vi "UHR-Fleezers Control (fpga) - 10.1.vi"() -> ()   [LabVIEW 2009]
doc: "UHR-Fleezers Instrument Control Code (fpga)"
uses:
  <vilib>/Platform/TimedLoop/XDataNode/XDataNode.xnode
  <vilib>/Platform/TimedLoop/XDataNode/loadlvalarms.vi
  <vilib>/Platform/TimedLoop/XDataNode/timing_clust.ctl
  <vilib>/Platform/TimedLoop/XDataNode/nitl_modes.ctl
  <vilib>/Platform/TimedLoop/XDataNode/wakeup.ctl
  <vilib>/eio/EIONode/EIONode.xnode
  <vilib>/rvi/eio/nirviEIOImplementation/nirviEIOImplementation.xnode
  <vilib>/rvi/eio/common/nirviEmuTemplateMethod_noerrors.vi
  <vilib>/rvi/eio/common/nirviEmuClasses.ctl
  <vilib>/eio/EIOMethodNode/EIOMethodNode.xnode
  <vilib>/rvi/eio/nirviEIOMethodImplementation/nirviEIOMethodImplementation.xnode
  <vilib>/rvi/DataTransferAndStorage/Container/XNode/niFpgaContainer.xnode
  <vilib>/rvi/interface/RandomDataEmulation/niFpgaRandomDataHandleErrors.vi
  <vilib>/rvi/interface/RandomDataEmulation/nirviRandomDataFPGAFIFO.vi
  <vilib>/rvi/DataTransferAndStorage/Container/Common/niFpgaContainerMethod.ctl
  <vilib>/rvi/DataTransferAndStorage/Container/Common/niFpgaTransferTypeControl.ctl
  <vilib>/addons/control/pid/fpga.llb/XNode/niFpgaPID.xnode
  <vilib>/Platform/TimedLoop/XDataNode/XDNodeRunTimeDep.lvlib
panel:
  in  "Tab Control":T1(tab)
  in  "AI1 X Scale":u16
  in  "Trap Pos FB Monitor T1 or T2":bool
  in  "Trap Pos FB Negate Action":bool
  in  "Trap Pos. FB SP":fxp<+/-,16,1>
  in  "Trap Pos. FB Reset":bool
  in  "Trap Pos to FIFO":bool
  in  "AI Averages":u16=1 min=1 step=1
  in  "AI1 Sets to FIFO":T2={"Set 1"=TRUE, "Set 2"=TRUE, "Set 3"=FALSE}
  in  "N of AI1 Int Acq Sets":i16=2 min=1 max=3 step=1
  out "Number of AI channels":i16
  out "AI Late Counter":u32
  in  "ai count":u32=400
  out "AI late?":bool
  in  "+ phase":bool
  in  "Phase count adjustment":i16
  out "Relative phase":i16
  in  "DMA buffer timeout":i32
  in  "AI to FIFO":bool
  out "BD1 Frequency Out 1":u64
  out "BD1 Frequency Out 2":u64
  in  "Force feedback":bool
  out "AI1 X Set 1":fxp<+/-,16,1>
  in  "Trap Pos. FB Gains":T3={"proportional gain (Kc)"=0.0, "integral gain (Kc*Ts/Ti)"=10.0, "derivative gain (Kc*Td/Ts)"=0.0} {"proportional gain (Kc)" format="%.11g"; "integral gain (Kc*Ts/Ti)" format="%.11g"; "derivative gain (Kc*Td/Ts)" format="%.11g"}
  in  "Trap Pos. FB Range":T4={"output high"=0.999969482421875, "output low"=-1.0}
  in  "Trap Pos. FB Mult Factor":i64=2
  in  "Trap Pos. FB Offset Factor":i64
  out "AI1 X Set 2":fxp<+/-,16,1>
  out "Trap Pos FB Action":i64
  in  "Tab Control 2":T5(tab)
  in  "Swap F1 and F2":bool
  in  "Freq or Amp switch first":bool=TRUE
  in  "Cont. Scan":bool
  in  "Abort scan":bool
  in  "Cycles per step":u64
  in  "Scan BD":bool
  in  "Number of scans":u16
  in  "Scan steps":u64
  in  "Scan freq.  increment":i64
  out "Scanning":bool
  in  "Start scan":bool
  in  "OSK Bd 1":bool
  in  "Reset Bd 1":bool
  in  "RD":bool
  in  "PMODE":bool
  in  "OSK Bd 2":bool
  in  "Reset Bd 2":bool
  in  "Direct RF Box \nCommunication":bool
  in  "Data BD 2":u8 format="%08b"
  in  "Data BD 1":u8 format="%08b"
  in  "Address":u8 format="%02x"
  in  "Update Data":bool
  in  "FPGA Controls\n RF Box":bool
  in  "Number Interlace Cycles":u8=2 min=1 max=3
  in  "Interlace Off Parameters":u8=1 min=1 max=3
  in  "Interlace ON/OFF":bool
  out "DIO Relative phase":i16
  in  "Phase count adjustment (DIO)":i16
  in  "+ phase (DIO)":bool
  out "DIO Late Counter":u32
  out "DIO Late?":bool
  in  "DIO count 1 (ticks)":u32=400
  in  "DIO count 2 (ticks)":u32=400
  in  "DIO count 3 (ticks)":u32=400
  out "AI2 Y Sum Set 2":i16
  out "AI2 Y Sum Set 1":i16
  in  "FB Gains Set 1":T6={"proportional gain (Kc)"=10, "integral gain (Kc*Ts/Ti)"=5, "derivative gain (Kc*Td/Ts)"=0}
  in  "FB Setpoint Set 1":i16 min=0 step=1
  in  "FB Reset Set 1":bool
  in  "FB On/Off Set 1":bool
  in  "FB Reset Set 2":bool
  in  "FB On/Off Set 2":bool
  in  "FB Setpoint Set 2":i16 min=0 step=1
  in  "FB Gains Set 2":T6={"proportional gain (Kc)"=10, "integral gain (Kc*Ts/Ti)"=5, "derivative gain (Kc*Td/Ts)"=0}
  in  "FB output range 2":cluster{"output high":i16, "output low":i16}={"output high"=3000, "output low"=0}
  in  "FB output range 1":cluster{"output high":i16, "output low":i16}={"output high"=3000, "output low"=0}
  out "Scan I":u64
  in  "Amp switch delay":u16=5
  in  "Freq switch delay":u16
  in  "BD 2 Amplitude 1":u16
  in  "BD 1 Amplitude 1":u16
  in  "BD 2 Frequency 1":u64
  in  "BD 1 Frequency 1":u64
  in  "BD 2 Amplitude 2":u16
  in  "BD 1 Amplitude 2":u16
  in  "BD 2 Frequency 2":u64
  in  "BD 1 Frequency 2":u64
  in  "BD 2 Amplitude 3":u16
  in  "BD 1 Amplitude 3":u16
  in  "BD 2 Frequency 3":u64
  in  "BD 1 Frequency 3":u64
  out "Numeric":i32
  out "AO2 2":i16
  out "AO1 2":i16
  in  "1D or 2D Scan?":bool
  in  "Abort scan (MCL)":bool
  in  "MCL Scan Axis":bool
  in  "Cont. Scan (MCL)":bool
  out "Scan I (MCL)":u64
  in  "Number of scans (MCL)":u16
  out "Scanning MCL":bool
  in  "Scan steps (MCL)":u64
  in  "Cycles per step (MCL)":u64
  in  "Scan freq.  increment (MCL)":i16
  in  "Start scan (MCL)":bool
  in  "AO2":i16
  in  "AO1":i16
  out "MCL Late Counter":u32
  out "MCL Late?":bool
  in  "MCL count":u32=800
  out "MCL Relative Phase":i16
  in  "Phase count adjustment (MCL)":i16
  in  "+ phase (MCL)":bool
  in  "APD2 Trigger on Edge?":bool=TRUE
  in  "APD1 Trigger on Edge?":bool=TRUE
  in  "APD Gate Operating Mode":u8 max=2 step=1
  in  "Invert APD Gate":bool
  in  "APD Gate OFF Count":u32=100
  in  "APD Gate ON Count":u32=300
  out "APD 1 Gate Late Counter":u32
  out "APD 1 Gate Late?":bool
  out "APD 1 Gate Relative Phase":i16
  in  "Phase count adjustment (APD 1 Gate)":i16
  in  "+ phase (APD 1 Gate)":bool
  out "APD 2 Counts 0":u32
  out "APD 2 Counts 1":u32
  out "APD 1 Counts 0":u32
  out "APD 1 Counts 1":u32
  out "APD out state":bool
  in  "APD 2 AO offset":i16
  in  "APD 1 AO offset":i16
  in  "APD 2 AO scale factor":i16=1
  in  "APD 1 AO scale factor":i16=1
  in  "APD to FIFO":bool
  in  "APD Acq Rate Count":u32=20000000
  out "APD Acq Late Counter":u32
  out "APD Acq Late?":bool
  out "APD Acq Relative Phase":i16
  in  "Phase Count Adjustment (APD Acq)":i16
  in  "+ phase (APD Acq)":bool
  in  "Phase count adjustment (APD 2 Gate)":i16
  out "APD 2 Gate Late Counter":u32
  out "APD 2 Gate Late?":bool
  out "APD 2 Gate Relative Phase":i16
  in  "+ phase (APD 2 Gate)":bool
  in  "Green Filter Flipper":bool
  out "Green FB Signals":T7
  in  "Green FB Count":u32=1200
  out "Green Late Counter":u32
  out "Green FB Late?":bool
  out "Green FB Relative Phase":i16
  in  "Phase count adjustment (Green FB)":i16=10
  in  "+ phase (Green FB)":bool
  out "Green FB Sum":i16
  in  "Green int current ON count adj":u32=150
  in  "Current Out":u16=30000
  in  "Green FB On/Off":bool
  in  "Green FB Setpoint":i16=250 min=0 step=1
  in  "Green FB Gains":T6={"proportional gain (Kc)"=10, "integral gain (Kc*Ts/Ti)"=5, "derivative gain (Kc*Td/Ts)"=0}
  in  "Green FB Reset":bool
  in  "Operating Mode 2":u8=2 max=2 step=1
  in  "Invert GI 2":bool
  in  "Green interlace OFF count 2":u32=900
  in  "Green interlace ON count 2":u32=300
  out "GI Late Counter 2":u32
  out "GI Late? 2":bool
  out "GI Relative phase 2":i16
  in  "Phase count adjustment (GI) 2":i16=20
  in  "+ phase (GI) 2":bool
  in  "Green interlace OFF count":u32=100
  out "GI Relative phase":i16
  in  "Phase count adjustment (GI)":i16
  in  "+ phase (GI)":bool
  out "GI Late?":bool
  in  "Green interlace ON count":u32=300
  out "GI Late Counter":u32
  in  "Invert GI":bool
  in  "Operating Mode":u8 max=2 step=1
  in  "Connector0/DIO9":bool
  in  "Connector1/DIO32":bool
  in  "Connector1/DIO33":bool
  in  "Connector1/DIO34":bool
  in  "Chassis2/Mod4/AO1":u16
  in  "Extra DO Counts":u32=40000
  # "Only one of these can be on\nat a time:"
  # "Raster Scan AOD"
  # "1 (X)"
  # "2 (Y)"
  # "IR Intensity Feedback (RF BD 1)"
  # "AO1 (Y)"
  # "2D"
  # "1D"
  # "AO2 (X)"
  # "APD AO for aligning"
  # "Detection Loop"
  # "Green fluorescent laser digital gate interlacing loop"
  # "0 Forced ON\n1 Forced OFF\n2 Interlacing"
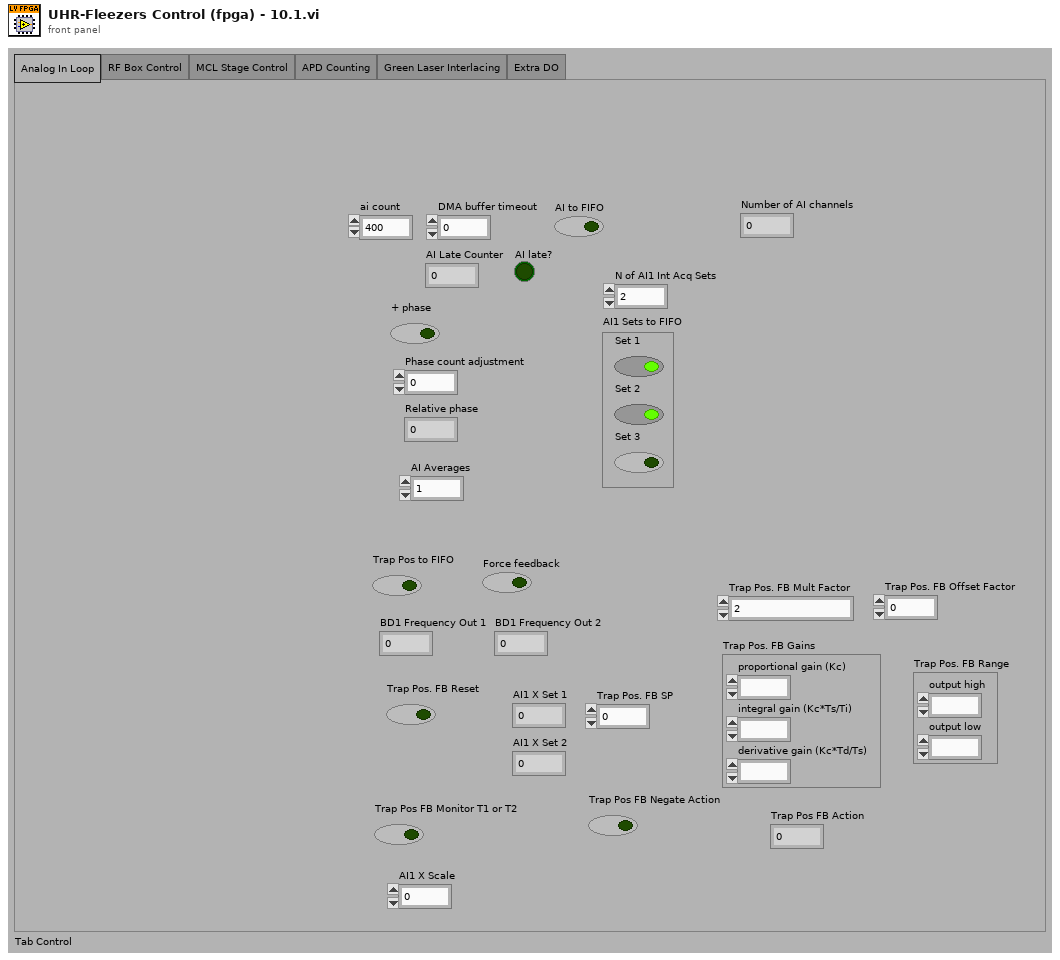
[diagram p1: front panel]
types:
  T1 = enum32{"Analog In Loop", "RF Box Control", "MCL Stage Control", "APD Counting", "Green Laser Interlacing", "Extra DO"}
  T2 = cluster{"Set 1":bool, "Set 2":bool, "Set 3":bool}
  T3 = cluster{"proportional gain (Kc)":fxp<+/-,16,8>, "integral gain (Kc*Ts/Ti)":fxp<+/-,16,8>, "derivative gain (Kc*Td/Ts)":fxp<+/-,16,8>}
  T4 = cluster{"output high":fxp<+/-,16,1>, "output low":fxp<+/-,16,1>}
  T5 = enum32{"Controls", "Interlacing Frequency and Amplitude Values"}
  T6 = cluster{"proportional gain (Kc)":i16, "integral gain (Kc*Ts/Ti)":i16, "derivative gain (Kc*Td/Ts)":i16}
  T7 = cluster{"Green FB Ch 0":i16, "Green FB Ch 1":i16, "Green FB Ch 2":i16}
  T8 = typedef "nirviEmuClasses.ctl" = enum16{"IO Read", "IO Write", "Method", "Property Read", "Property Write"}
  T9 = typedef "XDNodeRunTimeDep.lvlib/timing_clust.ctl" = cluster{"Expected End [f-1]":u64, "Actual End [f-1]":u64, "Finished Late? [f-1]":bool, "Expected End [i-1]":u64, "Actual End [i-1]":u64, "Finished Late? [i-1]":bool, "Expected Start [i]":u64, "Actual Start [i]":u64, "Expected Start [f]":u64, "Actual Start [f]":u64, "Source Name":string, "Structure Name":string, "Period":i64, "Deadline":i64, "Offset":i64, "Start":i64, "Priority":i32, "Timeout":i32, "Mode":T10, "Wakeup Reason":T11, "Error":errorcluster, "Source Type":string, "Secondary Source Type":string, "Global End Time":u64, "Global Start Time":u64, "Frame Duration":u64, "Iteration Duration":u64, "Assigned CPU":i32, "I/O Scan Engine Mode":u32}
  T10 = typedef "XDNodeRunTimeDep.lvlib/nitl_modes.ctl" = enum32{"No Change", "Process missed periods, maintain original phase", "Discard missed periods, maintain original phase", "Process missed periods, ignore original phase", "Discard missed periods, ignore original phase"}
  T11 = typedef "XDNodeRunTimeDep.lvlib/wakeup.ctl" = enum32{"Normal", "Aborted", "Asynchronous wakeup", "Timing source error", "Timed loop error", "Timeout"}
  T12 = typedef "niFpgaContainerMethod.ctl" = enum16{"Write", "Read", "Clear", "Get Number of Elements to Write", "Get Number of Elements to Read", "Enable", "Disable", "Flush and Disable", "Get Stream State"}
  T13 = typedef "niFpgaTransferTypeControl.ctl" = enum16{"Target-Scoped", "Host to Target - DMA", "Target to Host - DMA", "Peer to Peer Reader", "Peer to Peer Writer", "Bidirectional"}
  T14 = cluster{"Chassis2/Mod1/AI0":i16, "Chassis2/Mod1/AI1":i16, "Chassis2/Mod1/AI2":i16}
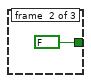
[diagram p2: hidden frame]
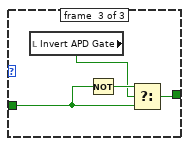
[diagram p3: hidden frame]
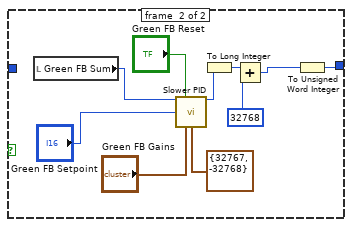
[diagram p4: hidden frame]
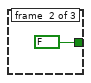
[diagram p5: hidden frame]
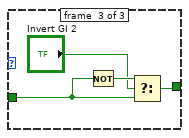
[diagram p6: hidden frame]
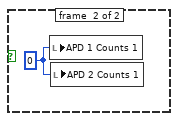
[diagram p7: hidden frame]
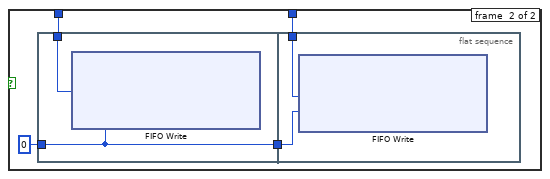
[diagram p8: hidden frame]
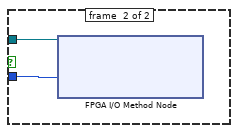
[diagram p9: hidden frame]
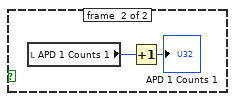
[diagram p10: hidden frame]
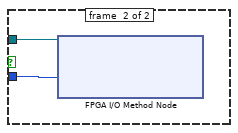
[diagram p11: hidden frame]
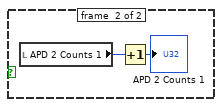
[diagram p12: hidden frame]
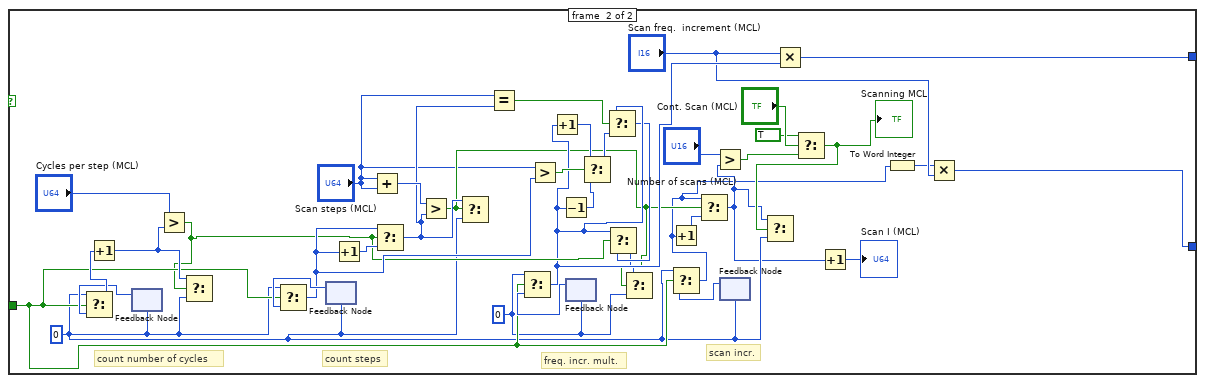
[diagram p13: hidden frame]
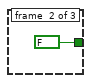
[diagram p14: hidden frame]
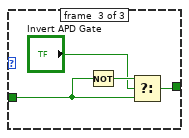
[diagram p15: hidden frame]
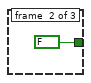
[diagram p16: hidden frame]
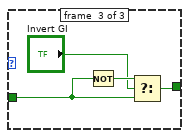
[diagram p17: hidden frame]
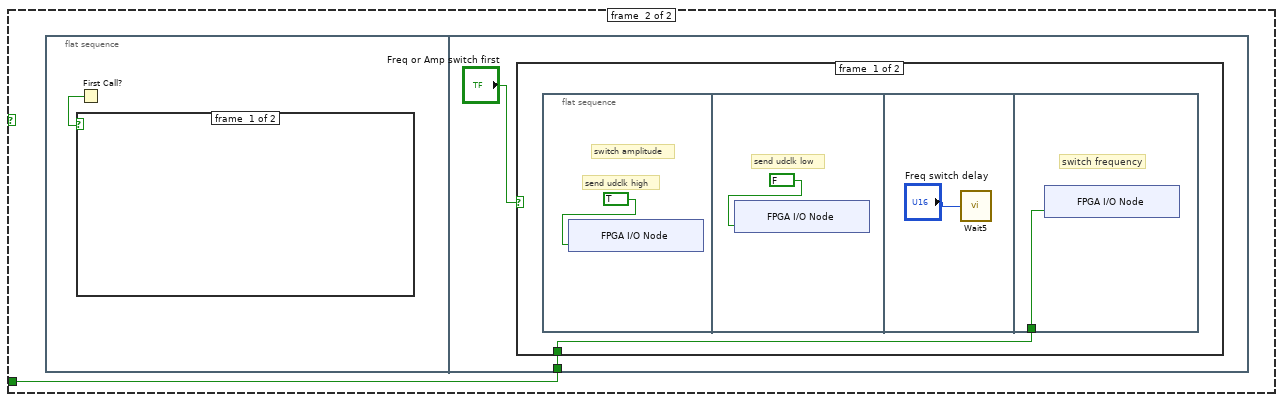
[diagram p18: hidden frame]
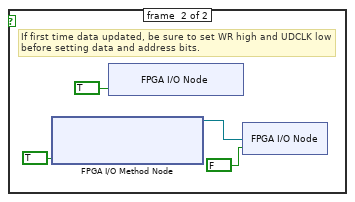
[diagram p19: hidden frame]
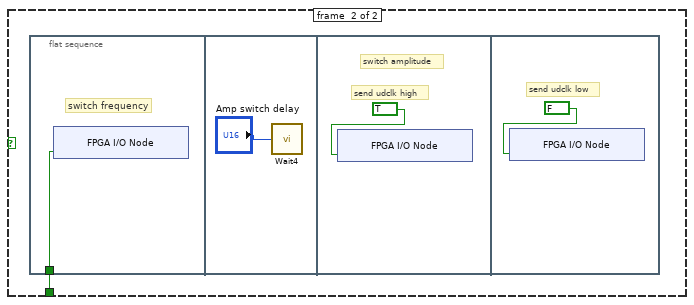
[diagram p20: hidden frame]
diagram:
  w2 = FALSE
  # "timing array current index"
  # "timing array"
  # "timing counter (phase adjusted here)"
  # "late counter"
  n1 = flat-sequence "FPGA initialization to do before running any of the loops" {
    tunnel: [u32 0 ("DIO count 3 (ticks)")] -> w1
    tunnel: [w10] -> _
    frame #0 {
      # "This is a kludge to let host programs know how many channels of data are in the DMA stream.  Set by hand."
      # "Start up expansion chassis early\nto avoid delays later"
      # "This pin controls udclk on the RF boards.\nWhen initially configuring the boards, this pin needs to be\nconfigured as a high impedance input.  Later it will be switched\nto an output."
      # "Initial setting of DIO data and \naddress to low (before reset).  \nThis needs to happen before the other\ncontrol method loops execute."
      n2 = xnode "FPGA I/O Node"("Chassis2/Mod4/AO0"=u16 0) -> ("Chassis2/Mod1/AI0"=w10:i16)  [unwired: 2 in, 2 out]
      n3 = xnode "FPGA I/O Method Node"("Enable"=FALSE) -> ()  [unwired: 1 in, 1 out]
      n4 = xnode "FPGA I/O Node"("Connector1/DIO0"=FALSE, "Connector1/DIO1"=FALSE, "Connector1/DIO2"=FALSE, "Connector1/DIO3"=FALSE, "Connector1/DIO4"=FALSE, "Connector1/DIO5"=FALSE, "Connector1/DIO6"=FALSE, "Connector1/DIO7"=FALSE, "Connector1/DIO8"=FALSE, "Connector1/DIO9"=FALSE, "Connector1/DIO10"=FALSE, "Connector1/DIO11"=FALSE, "Connector1/DIO12"=FALSE, "Connector1/DIO13"=FALSE, "Connector1/DIO15"=FALSE, "Connector1/DIO20"=FALSE, "Connector1/DIO21"=FALSE, "Connector1/DIO22"=FALSE, "Connector1/DIO23"=FALSE, "Connector1/DIO24"=FALSE, "Connector1/DIO25"=FALSE, "Connector1/DIO26"=FALSE, "Connector1/DIO27"=FALSE, "Connector1/DIO14"=FALSE) -> ()  [unwired: 24 in, 24 out]
      "Number of AI channels" <- i16 12 ("Number of AI channels")
    }
  }
  n5 = local read "AO1"() -> (w6:i16)
  n6 = local read "AO2"() -> (w5:i16)
  n7 = node-c288() -> (w4:T9)  [unwired: 1 in]
  n8 = while "APD 1 Counter" {
    tunnel: w1 -> [_]
    stop <- FALSE stop-if-true
    n9 = flat-sequence {
      frame #0 {
        n10 = case shown="False" "APD1 Trigger on Edge?" {
          tunnel: refnum<k21> "Connector0/DIO0" ("APD 1 DO") -> [w398 w423]
          tunnel: -1 ("Timeout") -> [w397 w422]
          frame #0 {
            n11 = xnode "FPGA I/O Method Node"("FPGA I/O In"=w398, "Timeout"=w397) -> ()  [unwired: 2 out]
          }
          frame #1 {
            n12 = xnode "FPGA I/O Method Node"("FPGA I/O In"=w423, "Timeout"=w422) -> ()  [unwired: 2 out]
          }
        }
      }
      frame #1 {
        n13 = local read "APD out state"() -> (w447:bool)
        n14 = case shown="False" w447 {
          frame #0 {
            n15 = local read "APD 1 Counts 0"() -> (w449:u32)
            n16 = Increment(x=w449) -> (x+1=→"APD 1 Counts 0":u32)
          }
          frame #1 {
            n17 = local read "APD 1 Counts 1"() -> (w451:u32)
            n18 = Increment(x=w451) -> (x+1=→"APD 1 Counts 1":u32)
          }
        }
      }
    }
  }
  n19 = while "APD 2 Counter" {
    tunnel: w1 -> [_]
    stop <- FALSE stop-if-true
    n20 = flat-sequence {
      frame #0 {
        n21 = case shown="False" "APD2 Trigger on Edge?" {
          tunnel: refnum<k21> "Connector0/DIO1" ("APD 2 DO") -> [w457 w482]
          tunnel: -1 ("Timeout") -> [w456 w481]
          frame #0 {
            n22 = xnode "FPGA I/O Method Node"("FPGA I/O In"=w457, "Timeout"=w456) -> ()  [unwired: 2 out]
          }
          frame #1 {
            n23 = xnode "FPGA I/O Method Node"("FPGA I/O In"=w482, "Timeout"=w481) -> ()  [unwired: 2 out]
          }
        }
      }
      frame #1 {
        n24 = local read "APD out state"() -> (w506:bool)
        n25 = case shown="False" w506 {
          frame #0 {
            n26 = local read "APD 2 Counts 0"() -> (w508:u32)
            n27 = Increment(x=w508) -> (x+1=→"APD 2 Counts 0":u32)
          }
          frame #1 {
            n28 = local read "APD 2 Counts 1"() -> (w510:u32)
            n29 = Increment(x=w510) -> (x+1=→"APD 2 Counts 1":u32)
          }
        }
      }
    }
  }
  n30 = while "APD 2 Gating" {
    shift-right: [w514] -> _
    shift-left: w1 -> [w519]
    shift-right: [w513] -> _
    shift-left: w2 -> [w511]
    stop <- FALSE stop-if-true
    n31 = flat-sequence {
      tunnel: w519 -> [w522]
      tunnel: [w523] -> w517
      tunnel: [w522] -> w515
      tunnel: [w521] -> w512
      tunnel: w511 -> [w521]
      tunnel: [w526] -> w518
      tunnel: w517 -> [w526]
      tunnel: [w525] -> w516
      tunnel: w515 -> [w525]
      tunnel: w512 -> [w524]
      tunnel: [w580] -> w514
      tunnel: w518 -> [w598]
      tunnel: w516 -> [w596]
      tunnel: [w585] -> w513
      frame #0 {
        n32 = call "Loop Timer8"("Count(Ticks)"=w522) -> ("Tick Count(Ticks)"=w523:u32)
      }
      frame #1 {
        # "(need 4 channels/APD)"
        n33 = xnode "FPGA I/O Node"("Connector0/DIO8"=w524, "Connector0/DIO9"=w524, "Connector0/DIO10"=w524, "Connector0/DIO11"=w524) -> ()  [unwired: 4 in, 4 out]
      }
      frame #2 {
        n34 = local read "APD Gate ON Count"() -> (w573:u32)
        n35 = local read "APD Gate OFF Count"() -> (w572:u32)
        n36 = feedback #1(TRUE) -> (w587:bool)
        n37 = feedback #2(w598) -> (w574:u32)
        n38 = Not(x=w587) -> (.not. x?=w584:bool)
        n39 = Subtract(x=w598, y=w574) -> (x-y=w597:u32)
        n40 = Select(t=w573, s=w584, f=w572) -> (s? t:f=w589:u32)
        n41 = Subtract(x=w597, y=w596) -> (x-y=w590:u32)
        n42 = Subtract(x=w589, y=w590) -> (x-y=w579:u32)
        n43 = Greater?(x=w590, y=u32 0) -> (0:w592:bool)
        "APD 2 Gate Late?" <- w592
        n44 = Boolean To (0,1)(Boolean="+ phase (APD 2 Gate)") -> (0, 1=w577:i16)
        n45 = Multiply(x=w577, y="Phase count adjustment (APD 2 Gate)") -> (x*y=w575:i16)
        n46 = feedback #3(u32 0) -> (w594:u32)
        n47 = Increment(x=w594) -> (x+1=w593:u32)
        n48 = Select(t=w593, s=w592, f=w594) -> (s? t:f=w591:u32)
        "APD 2 Gate Late Counter" <- w591
        n49 = Add(x=w579, y=w575) -> (x+y=w580:u32)
        n50 = feedback #4(i16 0) -> (w582:i16)
        n51 = Subtract(x=w582, y=w575) -> (x-y=w581:i16)
        "APD 2 Gate Relative Phase" <- w581
        n52 = local read "APD Gate Operating Mode"() -> (w571:u8)
        n53 = case shown="2" w571 {
          tunnel: [TRUE FALSE w604] -> w585
          tunnel: w587 -> [_ _ w602]
          frame #0 {
          }
          frame #1 {
          }
          frame #2 {
            n54 = local read "Invert APD Gate"() -> (w601:bool)
            n55 = Not(x=w602) -> (.not. x?=w603:bool)
            n56 = Select(t=w603, s=w601, f=w602) -> (s? t:f=w604:bool)
          }
        }
      }
    }
  }
  n57 = while "DAQ AI set 1" {
    shift-right: [w605] -> _
    shift-left: w1 -> [w610]
    stop <- FALSE stop-if-true
    n58 = flat-sequence {
      tunnel: w610 -> [w620]
      tunnel: [w621] -> w608
      tunnel: [w620] -> w607
      tunnel: [w631] -> w618
      tunnel: [w630] -> w617
      tunnel: [w629] -> w616
      tunnel: [w628] -> w615
      tunnel: [w627] -> w614
      tunnel: [w626] -> w613
      tunnel: [w625] -> w612
      tunnel: [w624] -> w611
      tunnel: [w623] -> w609
      tunnel: w608 -> [w623]
      tunnel: w607 -> [w622]
      tunnel: [w622] -> w606
      tunnel: [w817] -> w605
      tunnel: w618 -> [w852]
      tunnel: w617 -> [w808]
      tunnel: w616 -> [w809]
      tunnel: w615 -> [w851]
      tunnel: w614 -> [w840]
      tunnel: w613 -> [w839]
      tunnel: w612 -> [w838]
      tunnel: w611 -> [w837]
      tunnel: w609 -> [w834]
      tunnel: w606 -> [w831]
      frame #0 {
        n59 = call "Loop Timer3"("Count(Ticks)"=w620) -> ("Tick Count(Ticks)"=w621:u32)
      }
      frame #1 {
        n60 = xnode "FPGA I/O Node"("Connector1/DIO31"=TRUE ("Connector1/DIO33")) -> ("Connector0/AI0"=w631:i16, "Connector0/AI1"=w630:i16, "Connector0/AI2"=w629:i16, "Connector0/AI3"=w628:i16, "Connector0/AI4"=w627:i16, "Connector0/AI5"=w626:i16, "Connector0/AI6"=w625:i16, "Connector0/AI7"=w624:i16)  [unwired: 9 in, 9 out]
      }
      frame #2 {
        w812 = FALSE ("AI to FIFO")
        # "Adjust phase after data acquired if button pressed"
        n61 = feedback #5(i16 1) -> (w844:i16)
        n62 = Increment(x=w844) -> (x+1=w850:i16)
        n63 = Scale By Power Of 2(n="AI1 X Scale", x=w808) -> (x*2^n=w806:i16)
        n64 = Greater?(x=w850, y="N of AI1 Int Acq Sets") -> (0:w847:bool)
        n65 = Divide(x=w806, y=w809) -> (x/y=w805:fxp<+/-,16,1>)
        n66 = Select(t=i16 1, s=w847, f=w850) -> (s? t:f=w849:i16)
        n67 = feedback #6(w812) -> (w810:bool)
        n68 = feedback #7(w812) -> (w836:bool)
        n69 = case shown="1, Default" w844 {
          tunnel: w809 -> [w855 w890 _]
          tunnel: "AI1 Sets to FIFO" -> [w861 w896 w927]
          tunnel: [w859 w894 w926] -> w841
          tunnel: ["AI to FIFO" w893 w925] -> w835
          tunnel: w836 -> [_ w893 w925]
          tunnel: "DMA buffer timeout" -> [w860 w895 _]
          tunnel: ["Trap Pos to FIFO" w891 w924] -> w811
          tunnel: w810 -> [_ w891 w924]
          tunnel: w805 -> [w854 w889 _]
          frame #0 {
            n70 = Unbundle By Name(w861) -> ("Set 1"=w859:bool)
            n71 = Compound Arithmetic op=AND("Trap Pos to FIFO", w859, "AI to FIFO") -> (w857:bool)
            n72 = case shown="True" w857 {
              tunnel: w860 -> [_ w863]
              frame #0 {
              }
              frame #1 {
                n73 = local read "BD1 Frequency Out 1"() -> (w862:u64)
                n74 = xnode ("FIFO Method Node")("Element"=w862, "Timeout"=w863) -> ()  [unwired: 1 in, 2 out]
              }
            }
            "AI2 Y Sum Set 1" <- w855
            "AI1 X Set 1" <- w854
          }
          frame #1 {
            n75 = Unbundle By Name(w896) -> ("Set 2"=w894:bool)
            n76 = Compound Arithmetic op=AND(w891, w894, w893) -> (w892:bool)
            n77 = case shown="True" w892 {
              tunnel: w895 -> [_ w898]
              frame #0 {
              }
              frame #1 {
                n78 = local read "BD1 Frequency Out 2"() -> (w897:u64)
                n79 = xnode ("FIFO Method Node")("Element"=w897, "Timeout"=w898) -> ()  [unwired: 1 in, 2 out]
              }
            }
            "AI2 Y Sum Set 2" <- w890
            "AI1 X Set 2" <- w889
          }
          frame #2 {
            n80 = Unbundle By Name(w927) -> ("Set 3"=w926:bool)
          }
        }
        n81 = And(x=w841, y=w835) -> (x .and. y?=w843:bool)
        n82 = case shown="True" w843 {
          tunnel: w852 -> [_ w932]
          tunnel: w808 -> [_ w933]
          tunnel: w809 -> [_ w934]
          tunnel: w851 -> [_ w935]
          tunnel: w840 -> [_ w939]
          tunnel: w839 -> [_ w938]
          tunnel: w838 -> [_ w937]
          tunnel: w837 -> [_ w936]
          tunnel: "DMA buffer timeout" -> [_ w928]
          frame #0 {
          }
          frame #1 {
            n83 = Greater?(x="AI Averages", y=u16 1) -> (0:w930:bool)
            n84 = case shown="False" w930 {
              tunnel: w939 -> [w950 w1007]
              tunnel: w938 -> [w949 w1006]
              tunnel: w937 -> [w948 w1005]
              tunnel: w936 -> [w947 w1004]
              tunnel: w935 -> [w946 w1003]
              tunnel: w934 -> [w951 w1002]
              tunnel: w933 -> [w952 w1001]
              tunnel: w932 -> [w953 w1000]
              tunnel: "AI Averages" -> [_ w987]
              tunnel: w928 -> [w941 w984]
              frame #0 {
                n85 = Join Numbers(hi=w953, lo=w952) -> ((hi.lo)=w945:u32)
                n86 = Join Numbers(hi=w951, lo=w946) -> ((hi.lo)=w944:u32)
                n87 = Join Numbers(hi=w950, lo=w949) -> ((hi.lo)=w943:u32)
                n88 = Join Numbers(hi=w948, lo=w947) -> ((hi.lo)=w942:u32)
                n89 = Build Array(w945, w944, w943, w942) -> (w940:u32[])
                n90 = for {
                  tunnel: w940 -> [w955] mode=indexing
                  tunnel: w941 -> [w956]
                  n91 = To Unsigned Long Integer(number=w955) -> (unsigned 32bit integer=w954:u32)
                  n92 = xnode ("FIFO Write")("Element"=w954, "Timeout"=w956) -> ()  [unwired: 1 in, 2 out]
                }
              }
              frame #1 {
                w991 = u16 0
                n93 = To Long Integer(number=w1000) -> (32bit integer=w993:i32)
                n94 = To Long Integer(number=w1001) -> (32bit integer=w1010:i32)
                n95 = To Long Integer(number=w1002) -> (32bit integer=w1009:i32)
                n96 = To Long Integer(number=w1003) -> (32bit integer=w1008:i32)
                n97 = To Long Integer(number=w1007) -> (32bit integer=w999:i32)
                n98 = To Long Integer(number=w1006) -> (32bit integer=w998:i32)
                n99 = To Long Integer(number=w1005) -> (32bit integer=w997:i32)
                n100 = To Long Integer(number=w1004) -> (32bit integer=w996:i32)
                n101 = Build Array(w993, w1010, w1009, w1008, w999, w998, w997, w996) -> (w982:i32[])
                n102 = feedback #8(w982) -> (w995:i32[])
                n103 = Add(x=w982, y=w995) -> (x+y=w994:i32[])
                n104 = feedback #9(w991) -> (w989:u16)
                n105 = Increment(x=w989) -> (x+1=w986:u16)
                n106 = Equal?(x=w986, y=u16 1) -> (x = y?=w985:bool)
                n107 = Select(t=w982, s=w985, f=w994) -> (s? t:f=w983:i32[])
                n108 = Greater Or Equal?(x=w986, y=w987) -> (x >= y?=w988:bool)
                n109 = Select(t=w991, s=w988, f=w986) -> (s? t:f=w990:u16)
                n110 = case shown="True" w988 {
                  tunnel: w983 -> [_ w1012]
                  tunnel: w984 -> [_ w1011]
                  frame #0 {
                  }
                  frame #1 {
                    n111 = for {
                      tunnel: w1012 -> [w1014] mode=indexing
                      tunnel: w1011 -> [w1015]
                      n112 = To Unsigned Long Integer(number=w1014) -> (unsigned 32bit integer=w1013:u32)
                      n113 = xnode ("FIFO Write")("Element"=w1013, "Timeout"=w1015) -> ()  [unwired: 1 in, 2 out]
                    }
                  }
                }
              }
            }
          }
        }
        n114 = feedback #10(w834) -> (w833:u32)
        n115 = Subtract(x=w834, y=w833) -> (x-y=w832:u32)
        n116 = Subtract(x=w832, y=w831) -> (x-y=w828:u32)
        n117 = Subtract(x="ai count", y=w828) -> (x-y=w818:u32)
        n118 = Greater?(x=w828, y=u32 0) -> (0:w826:bool)
        "AI late?" <- w826
        n119 = xnode "I/O Node"("Connector1/DIO31"=FALSE ("Connector1/DIO34")) -> ()  [unwired: 1 in, 1 out]
        n120 = Boolean To (0,1)(Boolean="+ phase") -> (0, 1=w820:i16)
        n121 = feedback #11(u32 0) -> (w824:u32)
        n122 = Increment(x=w824) -> (x+1=w823:u32)
        n123 = Select(t=w823, s=w826, f=w824) -> (s? t:f=w825:u32)
        "AI Late Counter" <- w825
        n124 = Multiply(x=w820, y="Phase count adjustment") -> (x*y=w814:i16)
        n125 = feedback #12(i16 0) -> (w816:i16)
        n126 = Add(x=w818, y=w814) -> (x+y=w817:u32)
        n127 = Subtract(x=w816, y=w814) -> (x-y=w815:i16)
        "Relative phase" <- w815
      }
    }
  }
  n128 = while "RF box board DIO control: parallel communication" {
    shift-right: [w1060] -> _
    shift-left: w1 -> [w1059]
    shift-right: [w1058] -> _
    shift-left: FALSE ("Swap F1 and F2") -> [w1057]
    stop <- FALSE stop-if-true
    n129 = flat-sequence {
      tunnel: w1057 -> [w1064]
      tunnel: w1059 -> [w1062]
      tunnel: [w1064] -> w1056
      tunnel: [w1063] -> w1055
      tunnel: [w1062] -> w1054
      tunnel: [w1070] -> w1060
      tunnel: [w1069] -> w1058
      tunnel: w1056 -> [w1068]
      tunnel: w1055 -> [w1066]
      tunnel: w1054 -> [w1065]
      frame #0 {
        n130 = call "Loop Timer"("Count(Ticks)"=w1062) -> ("Tick Count(Ticks)"=w1063:u32)
      }
      frame #1 {
        n131 = flat-sequence {
          tunnel: ["FPGA Controls\n RF Box"] -> w1067
          tunnel: w1068 -> [w1071]
          tunnel: [w1220] -> w1070
          tunnel: [w1240] -> w1069
          tunnel: w1067 -> [w1239]
          tunnel: w1066 -> [w1233]
          tunnel: w1065 -> [w1230]
          frame #0 {
            n132 = case shown="True" "FPGA Controls\n RF Box" {
              tunnel: w1071 -> [_ w1073]
              frame #0 {
              }
              frame #1 {
                n133 = flat-sequence {
                  tunnel: w1073 -> [w1118]
                  frame #0 {
                    n134 = First Call?() -> (First Call?: T/F=w1074:bool)
                    n135 = case shown="True" w1074 {
                      frame #0 {
                      }
                      frame #1 {
                        # "If first time data updated, be sure to set WR high and UDCLK low\nbefore setting data and address bits."
                        n136 = xnode "FPGA I/O Method Node"("Enable"=TRUE) -> ("FPGA I/O Out"=w1076:refnum<k21>)  [unwired: 1 in]
                        n137 = xnode "FPGA I/O Node"("Connector1/DIO15"=TRUE) -> ()  [unwired: 1 in, 1 out]
                        n138 = xnode "FPGA I/O Node"("I/O Item"=FALSE ("Connector1/DIO30"), "FPGA I/O In"=w1076) -> ()  [unwired: 1 out]
                      }
                    }
                  }
                  frame #1 {
                    n139 = case shown="True" "Freq or Amp switch first" {
                      tunnel: w1118 -> [w1120 w1164]
                      frame #0 {
                        n140 = flat-sequence {
                          tunnel: w1120 -> [w1150]
                          frame #0 {
                            # "switch amplitude"
                            # "send udclk high"
                            n141 = xnode "FPGA I/O Node"("Connector1/DIO30"=TRUE ("Connector1/DIO15")) -> ()  [unwired: 1 in, 1 out]
                          }
                          frame #1 {
                            # "send udclk low"
                            n142 = xnode "FPGA I/O Node"("Connector1/DIO30"=FALSE ("Connector1/DIO15")) -> ()  [unwired: 1 in, 1 out]
                          }
                          frame #2 {
                            n143 = call "Wait5"("Count(Ticks)"="Freq switch delay") -> ()  [unwired: 1 out]
                          }
                          frame #3 {
                            # "switch frequency"
                            n144 = xnode "FPGA I/O Node"("Connector1/DIO36"=w1150) -> ()  [unwired: 1 in, 1 out]
                          }
                        }
                      }
                      frame #1 {
                        n145 = flat-sequence {
                          tunnel: w1164 -> [w1165]
                          frame #0 {
                            # "switch frequency"
                            n146 = xnode "FPGA I/O Node"("Connector1/DIO36"=w1165) -> ()  [unwired: 1 in, 1 out]
                          }
                          frame #1 {
                            n147 = call "Wait4"("Count(Ticks)"="Amp switch delay") -> ()  [unwired: 1 out]
                          }
                          frame #2 {
                            # "switch amplitude"
                            # "send udclk high"
                            n148 = xnode "FPGA I/O Node"("Connector1/DIO30"=TRUE ("Connector1/DIO15")) -> ()  [unwired: 1 in, 1 out]
                          }
                          frame #3 {
                            # "send udclk low"
                            n149 = xnode "FPGA I/O Node"("Connector1/DIO30"=FALSE ("Connector1/DIO15")) -> ()  [unwired: 1 in, 1 out]
                          }
                        }
                      }
                    }
                  }
                }
              }
            }
          }
          frame #1 {
            # "This is the prior cycle's on time"
            # "increment timing\nindex, reset to 0 if \nend of matrix"
            # "Reset to begginning (1) when number of cycles reached."
            # "timing index"
            # "build byte stacks for writing data\n(must correspond to addresses array constant)"
            # "Timing housekeeping"
            # "Adjust phase if late\n(maintains constant phase relationship between cycles)"
            n150 = feedback #13(u8 0 ("t")) -> (w1236:u8)
            n151 = Increment(x=w1236) -> (x+1=w1280:u8)
            n152 = Increment(x="Number Interlace Cycles") -> (x+1=w1275:u8)
            n153 = Equal?(x=w1280, y=w1275) -> (x = y?=w1282:bool)
            n154 = Select(t=u8 1, s=w1282, f=w1280) -> (s? t:f=w1235:u8)
            n155 = Increment(x=w1235) -> (x+1=w1277:u8)
            n156 = Equal?(x=w1277, y=w1275) -> (x = y?=w1278:bool)
            n157 = Select(t=u8 1, s=w1278, f=w1277) -> (s? t:f=w1274:u8)
            n158 = Select(t=w1274, s="Interlace ON/OFF", f="Interlace Off Parameters") -> (s? t:f=w1258:u8)
            n159 = case shown="1, Default" w1258 {
              tunnel: [w1357 "BD 1 Frequency 2" "BD 1 Frequency 3"] -> w1270
              tunnel: [w1356 "BD 2 Frequency 2" "BD 2 Frequency 3"] -> w1259
              tunnel: ["BD 2 Amplitude 1" "BD 2 Amplitude 2" "BD 2 Amplitude 3"] -> w1208
              tunnel: [w1345 w1473 "BD 1 Amplitude 3"] -> w1211
              frame #0 {
                w1352 = u64 0 ("f")
                # "Trap 1"
                n160 = local read "Scanning"() -> (w1358:bool)
                n161 = Or(x=w1358, y="Start scan") -> (x .or. y?=w1350:bool)
                n162 = Not(x="Abort scan") -> (.not. x?=w1348:bool)
                n163 = And(x=w1348, y=w1350) -> (x .and. y?=w1347:bool)
                n164 = case "For raster scanning" shown="False" w1347 {
                  tunnel: [u64 0 w1461] -> w1353
                  tunnel: "Start scan" -> [_ w1446]
                  frame #0 {
                    n165 = local write "Scanning"(FALSE ("scanning")) -> ()
                  }
                  frame #1 {
                    w1430 = i64 0
                    w1429 = u64 0
                    # "scan incr."
                    # "freq. incr. mult."
                    # "count steps"
                    # "count number of cycles"
                    n166 = feedback #14(w1429) -> (w1458:u64)
                    n167 = Select(t=w1429, s=w1446, f=w1458) -> (s? t:f=w1460:u64)
                    n168 = Increment(x=w1460) -> (x+1=w1457:u64)
                    n169 = Greater?(x="Cycles per step", y=w1457) -> (0:w1439:bool)
                    n170 = Select(t=w1457, s=w1439, f=w1429) -> (s? t:f=w1456:u64)
                    n171 = feedback #15(w1429) -> (w1455:u64)
                    n172 = Select(t=w1429, s=w1446, f=w1455) -> (s? t:f=w1450:u64)
                    n173 = Increment(x=w1450) -> (x+1=w1454:u64)
                    n174 = Add(x="Scan steps", y="Scan steps") -> (x+y=w1453:u64)
                    n175 = Select(t=w1450, s=w1439, f=w1454) -> (s? t:f=w1434:u64)
                    n176 = Greater?(x=w1453, y=w1434) -> (0:w1433:bool)
                    n177 = Select(t=w1434, s=w1433, f=w1429) -> (s? t:f=w1451:u64)
                    n178 = Equal?(x="Scan steps", y=w1434) -> (x = y?=w1438:bool)
                    n179 = Greater?(x="Scan steps", y=w1450) -> (0:w1449:bool)
                    n180 = feedback #16(w1430) -> (w1452:i64)
                    n181 = Select(t=w1430, s=w1446, f=w1452) -> (s? t:f=w1436:i64)
                    n182 = Increment(x=w1436) -> (x+1=w1448:i64)
                    n183 = Decrement(x=w1436) -> (x-1=w1447:i64)
                    n184 = Select(t=w1448, s=w1449, f=w1447) -> (s? t:f=w1437:i64)
                    n185 = Select(t=w1436, s=w1438, f=w1437) -> (s? t:f=w1435:i64)
                    n186 = Select(t=w1436, s=w1439, f=w1435) -> (s? t:f=w1431:i64)
                    n187 = Select(t=w1431, s=w1433, f=w1430) -> (s? t:f=w1432:i64)
                    n188 = feedback #17(w1429) -> (w1445:u64)
                    n189 = Select(t=w1429, s=w1446, f=w1445) -> (s? t:f=w1441:u64)
                    n190 = Increment(x=w1441) -> (x+1=w1442:u64)
                    n191 = Select(t=w1441, s=w1433, f=w1442) -> (s? t:f=w1440:u64)
                    n192 = Greater?(x="Number of scans", y=w1440) -> (0:w1426:bool)
                    n193 = Multiply(x="Scan freq.  increment", y=w1436) -> (x*y=w1461:i64)
                    n194 = Select(t=TRUE, s="Cont. Scan", f=w1426) -> (s? t:f=w1425:bool)
                    "Scanning" <- w1425
                    n195 = Select(t=w1440, s=w1425, f=w1429) -> (s? t:f=w1443:u64)
                    n196 = Increment(x=w1440) -> (x+1=→"Scan I":u64)
                  }
                }
                n197 = case "For position feedback" shown="True" "Force feedback" {
                  tunnel: [i64 0 w1376] -> w1342
                  frame #0 {
                  }
                  frame #1 {
                    n198 = case shown="False" "Trap Pos FB Monitor T1 or T2" {
                      tunnel: [w1383 w1384] -> w1370
                      frame #0 {
                        n199 = local read "AI1 X Set 2"() -> (w1383:fxp<+/-,16,1>)
                      }
                      frame #1 {
                        n200 = local read "AI1 X Set 1"() -> (w1384:fxp<+/-,16,1>)
                      }
                    }
                    n201 = xnode ("PID")("process variable"=w1370, "reset?"="Trap Pos. FB Reset", "setpoint"="Trap Pos. FB SP", "PID gains"="Trap Pos. FB Gains", "output range"="Trap Pos. FB Range") -> ("output"=w1374:fxp<+/-,16,1>)
                    n202 = Negate(x=w1374) -> (-x=w1373:fxp<+/-,17,2>)
                    n203 = Select(t=w1373, s="Trap Pos FB Negate Action", f=w1374) -> (s? t:f=w1368:fxp<+/-,17,2>)
                    n204 = Scale By Power Of 2(n=u32 15, x=u32 1) -> (x*2^n=w1365:u32)
                    n205 = Multiply(x=w1368, y=w1365) -> (x*y=w1364:fxp<+/-,17,17>)
                    n206 = To Quad Integer(1:w1364) -> (0:w1379:i64)
                    "Trap Pos FB Action" <- w1379
                    n207 = Multiply(x=w1379, y="Trap Pos. FB Mult Factor") -> (x*y=w1377:i64)
                    n208 = Add(x=w1377, y="Trap Pos. FB Offset Factor") -> (x+y=w1376:i64)
                  }
                }
                n209 = case "For intensity feedback" shown="True" "FB On/Off Set 1" {
                  tunnel: "BD 1 Amplitude 1" -> [w1463 _]
                  tunnel: [w1463 w1464] -> w1345
                  frame #0 {
                  }
                  frame #1 {
                    n210 = local read "AI2 Y Sum Set 1"() -> (w1466:i16)
                    n211 = call "Slower PID.vi"("process variable"=w1466, "reset?"="FB Reset Set 1", "setpoint"="FB Setpoint Set 1", "PID gains (x 2^8)"="FB Gains Set 1", "output range"="FB output range 1") -> ("output"=w1469:i16)  [unwired: 10 out]
                    n212 = To Unsigned Word Integer(number=w1469) -> (unsigned 16bit integer=w1464:u16)
                  }
                }
                n213 = Select(t=w1352, s="Scan BD", f=w1353) -> (s? t:f=w1351:u64)
                n214 = Select(t=w1353, s="Scan BD", f=w1352) -> (s? t:f=w1354:u64)
                n215 = Add(x=w1351, y="BD 2 Frequency 1") -> (x+y=w1356:u64)
                n216 = Compound Arithmetic op=ADD("BD 1 Frequency 1", w1342, w1354) -> (w1357:u64)
                "BD1 Frequency Out 1" <- w1357
              }
              frame #1 {
                # "Trap 2"
                n217 = case shown="True" "FB On/Off Set 2" {
                  tunnel: [w1477 w1478] -> w1473
                  tunnel: "BD 1 Amplitude 2" -> [w1477 _]
                  frame #0 {
                  }
                  frame #1 {
                    n218 = local read "AI2 Y Sum Set 2"() -> (w1483:i16)
                    n219 = call "Slower PID.vi"("process variable"=w1483, "reset?"="FB Reset Set 2", "setpoint"="FB Setpoint Set 2", "PID gains (x 2^8)"="FB Gains Set 2", "output range"="FB output range 2") -> ("output"=w1480:i16)  [unwired: 10 out]
                    n220 = To Unsigned Word Integer(number=w1480) -> (unsigned 16bit integer=w1478:u16)
                  }
                }
                "BD1 Frequency Out 2" <- "BD 1 Frequency 2"
              }
              frame #2 {
                # "Fluorescence period"
              }
            }
            n221 = feedback #18(w1233) -> (w1232:u32)
            n222 = Subtract(x=w1233, y=w1232) -> (x-y=w1231:u32)
            n223 = Select(t=w1235, s="Interlace ON/OFF", f="Interlace Off Parameters") -> (s? t:f=w1273:u8)
            n224 = Subtract "The error"(x=w1231, y=w1230) -> (x-y=w1228:u32)
            n225 = case shown="3" w1273 {
              tunnel: ["DIO count 1 (ticks)" "DIO count 2 (ticks)" "DIO count 3 (ticks)"] -> w1229
              frame #0 {
              }
              frame #1 {
              }
              frame #2 {
              }
            }
            n226 = Greater?(x=w1228, y=u32 0) -> (0:w1223:bool)
            "DIO Late?" <- w1223
            n227 = feedback #19(u32 0) -> (w1225:u32)
            n228 = Increment(x=w1225) -> (x+1=w1224:u32)
            n229 = Select(t=w1224, s=w1223, f=w1225) -> (s? t:f=w1226:u32)
            "DIO Late Counter" <- w1226
            n230 = Subtract(x=w1229, y=w1228) -> (x-y=w1221:u32)
            n231 = Boolean To (0,1)(Boolean="+ phase (DIO)") -> (0, 1=w1218:i16)
            n232 = Multiply(x=w1218, y="Phase count adjustment (DIO)") -> (x*y=w1214:i16)
            n233 = feedback #20(i16 0) -> (w1216:i16)
            n234 = Subtract(x=w1216, y=w1214) -> (x-y=w1215:i16)
            "DIO Relative phase" <- w1215
            n235 = Split Number(x=w1270) -> (hi(x)=w1269:u32, lo(x)=w1268:u32)
            n236 = Split Number(x=w1259) -> (hi(x)=w1264:u32, lo(x)=w1263:u32)
            n237 = Split Number(x=w1269) -> (lo(x)=w1267:u16)  [unwired: 1 out]
            n238 = Split Number(x=w1268) -> (hi(x)=w1266:u16, lo(x)=w1265:u16)
            n239 = Split Number(x=w1264) -> (lo(x)=w1262:u16)  [unwired: 1 out]
            n240 = Split Number(x=w1263) -> (hi(x)=w1261:u16, lo(x)=w1260:u16)
            n241 = Split Number(x=w1211) -> (hi(x)=w1213:u8, lo(x)=w1212:u8)
            n242 = Split Number(x=w1208) -> (hi(x)=w1210:u8, lo(x)=w1209:u8)
            n243 = Add(x=w1221, y=w1214) -> (x+y=w1220:u32)
            n244 = Split Number(x=w1267) -> (hi(x)=w1257:u8, lo(x)=w1256:u8)
            n245 = Split Number(x=w1266) -> (hi(x)=w1255:u8, lo(x)=w1254:u8)
            n246 = Split Number(x=w1262) -> (hi(x)=w1250:u8, lo(x)=w1249:u8)
            n247 = Split Number(x=w1265) -> (hi(x)=w1253:u8, lo(x)=w1252:u8)
            n248 = Split Number(x=w1261) -> (hi(x)=w1248:u8, lo(x)=w1247:u8)
            n249 = Split Number(x=w1260) -> (hi(x)=w1246:u8, lo(x)=w1245:u8)
            n250 = Build Array "BD 1 A Stack"(w1213, w1212) -> (w1242:u8[])
            n251 = Build Array "BD 2 A Stack"(w1210, w1209) -> (w1241:u8[])
            n252 = Build Array "BD 1 nu Stack"(w1257, w1256, w1255, w1254, w1253, w1252) -> (w1251:u8[])
            n253 = Build Array "BD 2 nu Stack"(w1250, w1249, w1248, w1247, w1246, w1245) -> (w1244:u8[])
            n254 = case shown="2" w1258 {
              tunnel: [w1334 w1337] -> w1240
              tunnel: [u8 10 u8 4] -> w1243
              tunnel: "Swap F1 and F2" -> [w1335 w1337]
              frame #0 {
                # "F2"
                n255 = Not(x=w1335) -> (.not. x?=w1334:bool)
              }
              frame #1 {
                # "low chooses F1"
                # "F1"
              }
            }
            n256 = case "If FPGA is controlling (toggling) RF synth" shown="True" w1239 {
              tunnel: w1251 -> [_ w1287]
              tunnel: w1244 -> [_ w1286]
              tunnel: w1243 -> [_ w1285]
              tunnel: w1242 -> [_ w1284]
              tunnel: w1241 -> [_ w1283]
              frame #0 {
              }
              frame #1 {
                # "Write next amp.\n(wait until beginning of next loop iteration to update)"
                n257 = flat-sequence "Update the next F1 and F2 frequency value (the actual frequency won't change until FSK is switched).\nThen load the next amplitude value into buffer, but don't update it until the next cycle." {
                  tunnel: w1287 -> [w1290]
                  tunnel: w1286 -> [w1289]
                  tunnel: w1285 -> [w1288]
                  tunnel: w1284 -> [w1327]
                  tunnel: w1283 -> [w1326]
                  frame #0 {
                    n258 = for {
                      tunnel: w1290 -> [w1296] mode=indexing
                      tunnel: w1289 -> [w1295] mode=indexing
                      tunnel: w1288 -> [w1293]
                      i -> [w1294]
                      # "Write next freq."
                      n259 = To Unsigned Byte Integer(number=w1294) -> (unsigned 8bit integer=w1291:u8)
                      n260 = Add(x=w1293, y=w1291) -> (x+y=w1292:u8)
                      n261 = call "write to RF synth bd.vi"("Address Byte"=w1292, "BD 2 Byte"=w1295, "BD 1 Byte"=w1296) -> ()
                    }
                  }
                  frame #1 {
                    # "send udclk high"
                    n262 = xnode "FPGA I/O Node"("Connector1/DIO30"=TRUE ("Connector1/DIO15")) -> ()  [unwired: 1 in, 1 out]
                  }
                  frame #2 {
                    n263 = xnode "FPGA I/O Node"("Connector1/DIO30"=FALSE ("Connector1/DIO15")) -> ()  [unwired: 1 in, 1 out]
                  }
                  frame #3 {
                    n264 = for {
                      tunnel: w1327 -> [w1333] mode=indexing
                      tunnel: w1326 -> [w1332] mode=indexing
                      tunnel: u8 33 -> [w1330]
                      i -> [w1331]
                      n265 = To Unsigned Byte Integer(number=w1331) -> (unsigned 8bit integer=w1328:u8)
                      n266 = Add(x=w1330, y=w1328) -> (x+y=w1329:u8)
                      n267 = call "write to RF synth bd.vi"("Address Byte"=w1329, "BD 2 Byte"=w1332, "BD 1 Byte"=w1333) -> ()
                    }
                  }
                }
              }
            }
          }
        }
      }
    }
  }
  n268 = while "MCL stage control" {
    shift-right: [w1504] -> _
    shift-left: w1 -> [w1507]
    shift-right: [w1497] -> _
    shift-left: w6 -> [w1494]
    shift-right: [w1496] -> _
    shift-left: w5 -> [w1492]
    i -> [w1491]
    stop <- FALSE stop-if-true
    n269 = flat-sequence {
      tunnel: w1507 -> [w1511]
      tunnel: [w1512] -> w1503
      tunnel: [w1511] -> w1501
      tunnel: [w1510] -> w1495
      tunnel: w1494 -> [w1510]
      tunnel: [w1509] -> w1493
      tunnel: w1492 -> [w1509]
      tunnel: w1503 -> [w1516]
      tunnel: [w1516] -> w1502
      tunnel: w1501 -> [w1515]
      tunnel: [w1515] -> w1500
      tunnel: w1495 -> [w1514]
      tunnel: w1493 -> [w1513]
      tunnel: [w1514] -> w1490
      tunnel: [w1513] -> w1489
      tunnel: w1502 -> [w1550]
      tunnel: w1500 -> [w1549]
      tunnel: [w1550] -> w1506
      tunnel: [w1549] -> w1505
      tunnel: [w1548] -> w1499
      tunnel: [w1547] -> w1498
      tunnel: w1490 -> [w1542]
      tunnel: w1489 -> [w1541]
      tunnel: [w1614] -> w1504
      tunnel: w1506 -> [w1628]
      tunnel: w1505 -> [w1625]
      tunnel: w1499 -> [w1617]
      tunnel: w1498 -> [w1616]
      tunnel: [w1617] -> w1497
      tunnel: [w1616] -> w1496
      frame #0 {
        n270 = call "Loop Timer5"("Count(Ticks)"=w1511) -> ("Tick Count(Ticks)"=w1512:u32)
      }
      frame #1 {
        n271 = xnode "FPGA I/O Node"("Connector0/AO1"=w1514, "Connector0/AO2"=w1513) -> ()  [unwired: 2 in, 2 out]
      }
      frame #2 {
        n272 = local read "Scanning MCL"() -> (w1562:bool)
        n273 = Or(x=w1562, y="Start scan (MCL)") -> (x .or. y?=w1557:bool)
        n274 = Not(x="Abort scan (MCL)") -> (.not. x?=w1555:bool)
        n275 = And(x=w1555, y=w1557) -> (x .and. y?=w1554:bool)
        n276 = case "Raster scan" shown="True" w1554 {
          tunnel: [w1563 w1606] -> w1559
          tunnel: "Start scan (MCL)" -> [_ w1591]
          tunnel: [w1563 w1567] -> w1543
          frame #0 {
            w1563 = i16 0
            n277 = local write "Scanning MCL"(FALSE ("scanning")) -> ()
          }
          frame #1 {
            w1577 = i16 0
            w1576 = u64 0
            # "scan incr."
            # "freq. incr. mult."
            # "count steps"
            # "count number of cycles"
            n278 = feedback #21(w1576) -> (w1603:u64)
            n279 = Select(t=w1576, s=w1591, f=w1603) -> (s? t:f=w1605:u64)
            n280 = Increment(x=w1605) -> (x+1=w1602:u64)
            n281 = Greater?(x="Cycles per step (MCL)", y=w1602) -> (0:w1586:bool)
            n282 = Select(t=w1602, s=w1586, f=w1576) -> (s? t:f=w1601:u64)
            n283 = feedback #22(w1576) -> (w1600:u64)
            n284 = Select(t=w1576, s=w1591, f=w1600) -> (s? t:f=w1595:u64)
            n285 = Increment(x=w1595) -> (x+1=w1599:u64)
            n286 = Add(x="Scan steps (MCL)", y="Scan steps (MCL)") -> (x+y=w1598:u64)
            n287 = Select(t=w1595, s=w1586, f=w1599) -> (s? t:f=w1581:u64)
            n288 = Greater?(x=w1598, y=w1581) -> (0:w1580:bool)
            n289 = Select(t=w1581, s=w1580, f=w1576) -> (s? t:f=w1596:u64)
            n290 = Equal?(x="Scan steps (MCL)", y=w1581) -> (x = y?=w1585:bool)
            n291 = Greater?(x="Scan steps (MCL)", y=w1595) -> (0:w1594:bool)
            n292 = feedback #23(w1577) -> (w1597:i16)
            n293 = Select(t=w1577, s=w1591, f=w1597) -> (s? t:f=w1583:i16)
            n294 = Increment(x=w1583) -> (x+1=w1593:i16)
            n295 = Decrement(x=w1583) -> (x-1=w1592:i16)
            n296 = Select(t=w1593, s=w1594, f=w1592) -> (s? t:f=w1584:i16)
            n297 = Select(t=w1583, s=w1585, f=w1584) -> (s? t:f=w1582:i16)
            n298 = Select(t=w1583, s=w1586, f=w1582) -> (s? t:f=w1578:i16)
            n299 = Select(t=w1578, s=w1580, f=w1577) -> (s? t:f=w1579:i16)
            n300 = feedback #24(w1576) -> (w1590:u64)
            n301 = Select(t=w1576, s=w1591, f=w1590) -> (s? t:f=w1565:u64)
            n302 = Increment(x=w1565) -> (x+1=w1587:u64)
            n303 = Select(t=w1565, s=w1580, f=w1587) -> (s? t:f=w1566:u64)
            n304 = Greater?(x="Number of scans (MCL)", y=w1566) -> (0:w1573:bool)
            n305 = Multiply(x="Scan freq.  increment (MCL)", y=w1583) -> (x*y=w1606:i16)
            n306 = Select(t=TRUE, s="Cont. Scan (MCL)", f=w1573) -> (s? t:f=w1572:bool)
            "Scanning MCL" <- w1572
            n307 = Select(t=w1566, s=w1572, f=w1576) -> (s? t:f=w1588:u64)
            n308 = Increment(x=w1566) -> (x+1=→"Scan I (MCL)":u64)
            n309 = To Word Integer(number=w1565) -> (16bit integer=w1568:i16)
            n310 = Multiply(x=w1568, y="Scan freq.  increment (MCL)") -> (x*y=w1567:i16)
          }
        }
        n311 = Select(t=w1543, s="1D or 2D Scan?", f=i16 0) -> (s? t:f=w1544:i16)
        n312 = Select(t=w1544, s="MCL Scan Axis", f=w1559) -> (s? t:f=w1558:i16)
        n313 = Select(t=w1559, s="MCL Scan Axis", f=w1544) -> (s? t:f=w1560:i16)
        n314 = Add(x=w1558, y="AO2") -> (x+y=w1547:i16)
        n315 = Add(x="AO1", y=w1560) -> (x+y=w1548:i16)
        "AO1 2" <- w1542
        "AO2 2" <- w1541
      }
      frame #3 {
        n316 = feedback #25(w1628) -> (w1627:u32)
        n317 = Boolean To (0,1)(Boolean="+ phase (MCL)") -> (0, 1=w1612:i16)
        n318 = Subtract(x=w1628, y=w1627) -> (x-y=w1626:u32)
        n319 = Multiply(x=w1612, y="Phase count adjustment (MCL)") -> (x*y=w1608:i16)
        n320 = Subtract(x=w1626, y=w1625) -> (x-y=w1623:u32)
        n321 = Subtract(x="MCL count", y=w1623) -> (x-y=w1610:u32)
        n322 = feedback #26(i16 0) -> (w1609:i16)
        n323 = Subtract(x=w1609, y=w1608) -> (x-y=w1607:i16)
        "MCL Relative Phase" <- w1607
        n324 = Greater?(x=w1623, y=u32 0) -> (0:w1622:bool)
        "MCL Late?" <- w1622
        n325 = Add(x=w1610, y=w1608) -> (x+y=w1614:u32)
        n326 = feedback #27(u32 0) -> (w1620:u32)
        n327 = Increment(x=w1620) -> (x+1=w1619:u32)
        n328 = Select(t=w1619, s=w1622, f=w1620) -> (s? t:f=w1621:u32)
        "MCL Late Counter" <- w1621
      }
    }
    "Numeric" <- w1491
  }
  n329 = while "APD 1 Gating" {
    shift-right: [w1633] -> _
    shift-left: w1 -> [w1638]
    shift-right: [w1632] -> _
    shift-left: w2 -> [w1630]
    stop <- FALSE stop-if-true
    n330 = flat-sequence {
      tunnel: w1638 -> [w1641]
      tunnel: [w1642] -> w1636
      tunnel: [w1641] -> w1634
      tunnel: [w1640] -> w1631
      tunnel: w1630 -> [w1640]
      tunnel: [w1645] -> w1637
      tunnel: w1636 -> [w1645]
      tunnel: [w1644] -> w1635
      tunnel: w1634 -> [w1644]
      tunnel: w1631 -> [w1643]
      tunnel: [w1695] -> w1633
      tunnel: w1637 -> [w1717]
      tunnel: w1635 -> [w1714]
      tunnel: [w1700] -> w1632
      frame #0 {
        n331 = call "Loop Timer7"("Count(Ticks)"=w1641) -> ("Tick Count(Ticks)"=w1642:u32)
      }
      frame #1 {
        # "(need 4 channels/APD)"
        n332 = xnode "FPGA I/O Node"("Connector0/DIO4"=w1643, "Connector0/DIO5"=w1643, "Connector0/DIO6"=w1643, "Connector0/DIO7"=w1643) -> ()  [unwired: 4 in, 4 out]
      }
      frame #2 {
        n333 = feedback #28(TRUE) -> (w1703:bool)
        n334 = feedback #29(w1717) -> (w1716:u32)
        n335 = Not(x=w1703) -> (.not. x?=w1699:bool)
        n336 = Subtract(x=w1717, y=w1716) -> (x-y=w1715:u32)
        n337 = Select(t="APD Gate ON Count", s=w1699, f="APD Gate OFF Count") -> (s? t:f=w1705:u32)
        n338 = Subtract(x=w1715, y=w1714) -> (x-y=w1706:u32)
        n339 = Subtract(x=w1705, y=w1706) -> (x-y=w1694:u32)
        n340 = Greater?(x=w1706, y=u32 0) -> (0:w1710:bool)
        "APD 1 Gate Late?" <- w1710
        n341 = Boolean To (0,1)(Boolean="+ phase (APD 1 Gate)") -> (0, 1=w1692:i16)
        n342 = Multiply(x=w1692, y="Phase count adjustment (APD 1 Gate)") -> (x*y=w1690:i16)
        n343 = feedback #30(u32 0) -> (w1712:u32)
        n344 = Increment(x=w1712) -> (x+1=w1711:u32)
        n345 = Select(t=w1711, s=w1710, f=w1712) -> (s? t:f=w1709:u32)
        "APD 1 Gate Late Counter" <- w1709
        n346 = Add(x=w1694, y=w1690) -> (x+y=w1695:u32)
        n347 = feedback #31(i16 0) -> (w1697:i16)
        n348 = Subtract(x=w1697, y=w1690) -> (x-y=w1696:i16)
        "APD 1 Gate Relative Phase" <- w1696
        n349 = case shown="2" "APD Gate Operating Mode" {
          tunnel: [TRUE FALSE w1723] -> w1700
          tunnel: w1703 -> [_ _ w1720]
          frame #0 {
          }
          frame #1 {
          }
          frame #2 {
            n350 = Not(x=w1720) -> (.not. x?=w1722:bool)
            n351 = Select(t=w1722, s="Invert APD Gate", f=w1720) -> (s? t:f=w1723:bool)
          }
        }
      }
    }
  }
  n352 = while "RF box board direct communication loop" {
    tunnel: w1 -> [_]
    stop <- FALSE stop-if-true
    n353 = case "Whether to use direct communication method (only use one method at a time)" shown="True" "Direct RF Box \nCommunication" {
      frame #0 {
      }
      frame #1 {
        n354 = case shown="True" "Update Data" {
          frame #0 {
          }
          frame #1 {
            n355 = flat-sequence {
              frame #0 {
                n356 = First Call?() -> (First Call?: T/F=w1727:bool)
                n357 = case shown="True" w1727 {
                  frame #0 {
                  }
                  frame #1 {
                    # "If first time data updated, be sure to set WR high\nbefore setting data and address bits."
                    n358 = flat-sequence {
                      frame #0 {
                        n359 = xnode "FPGA I/O Node"("Connector1/DIO15"=TRUE) -> ()  [unwired: 1 in, 1 out]
                      }
                      frame #1 {
                        n360 = call "Wait"("Count(Ticks)"=u8 40 ("DO Delay 3 (Ticks)")) -> ()  [unwired: 1 out]
                      }
                    }
                  }
                }
              }
              frame #1 {
                n361 = Number To Boolean Array(number="Address") -> (Boolean array=w1789:bool[])
                n362 = Number To Boolean Array(number="Data BD 1") -> (Boolean array=w1790:bool[])
                n363 = Number To Boolean Array(number="Data BD 2") -> (Boolean array=w1759:bool[])
                n364 = Index Array(array=w1790, index=7) -> (element=w1774:bool)
                n365 = Index Array(array=w1790, index=6) -> (element=w1773:bool)
                n366 = Index Array(array=w1790, index=5) -> (element=w1772:bool)
                n367 = Index Array(array=w1790, index=4) -> (element=w1771:bool)
                n368 = Index Array(array=w1790, index=3) -> (element=w1770:bool)
                n369 = Index Array(array=w1790, index=2) -> (element=w1769:bool)
                n370 = Index Array(array=w1790, index=1) -> (element=w1768:bool)
                n371 = Index Array(array=w1790, index=0) -> (element=w1767:bool)
                n372 = Index Array(array=w1789, index=5) -> (element=w1766:bool)
                n373 = Index Array(array=w1789, index=4) -> (element=w1765:bool)
                n374 = Index Array(array=w1789, index=3) -> (element=w1764:bool)
                n375 = Index Array(array=w1789, index=2) -> (element=w1763:bool)
                n376 = Index Array(array=w1789, index=1) -> (element=w1762:bool)
                n377 = Index Array(array=w1789, index=0) -> (element=w1761:bool)
                n378 = Index Array(array=w1759, index=7) -> (element=w1750:bool)
                n379 = Index Array(array=w1759, index=6) -> (element=w1749:bool)
                n380 = Index Array(array=w1759, index=5) -> (element=w1748:bool)
                n381 = Index Array(array=w1759, index=4) -> (element=w1747:bool)
                n382 = Index Array(array=w1759, index=3) -> (element=w1746:bool)
                n383 = Index Array(array=w1759, index=2) -> (element=w1745:bool)
                n384 = Index Array(array=w1759, index=1) -> (element=w1744:bool)
                n385 = Index Array(array=w1759, index=0) -> (element=w1743:bool)
                n386 = xnode "FPGA I/O Node"("Connector1/DIO0"=w1774, "Connector1/DIO1"=w1773, "Connector1/DIO2"=w1772, "Connector1/DIO3"=w1771, "Connector1/DIO4"=w1770, "Connector1/DIO5"=w1769, "Connector1/DIO6"=w1768, "Connector1/DIO7"=w1767, "Connector1/DIO8"=w1766, "Connector1/DIO9"=w1765, "Connector1/DIO10"=w1764, "Connector1/DIO11"=w1763, "Connector1/DIO12"=w1762, "Connector1/DIO13"=w1761, "Connector1/DIO20"=w1750, "Connector1/DIO21"=w1749, "Connector1/DIO22"=w1748, "Connector1/DIO23"=w1747, "Connector1/DIO24"=w1746, "Connector1/DIO25"=w1745, "Connector1/DIO26"=w1744, "Connector1/DIO27"=w1743) -> ()  [unwired: 22 in, 22 out]
              }
              frame #2 {
                # "wait and then apply write signal"
                n387 = call "Wait2"("Count(Ticks)"=u8 40 ("DO Delay 1 (Ticks)")) -> ()  [unwired: 1 out]
              }
              frame #3 {
                # "sending bit low writes data to board buffer"
                n388 = xnode "FPGA I/O Node"("Connector1/DIO15"=FALSE) -> ()  [unwired: 1 in, 1 out]
              }
              frame #4 {
                # "wait then return write signal"
                n389 = call "Wait3"("Count(Ticks)"=u8 40 ("DO Delay 2 (Ticks)")) -> ()  [unwired: 1 out]
              }
              frame #5 {
                # "sending bit high makes ready to\nwrite more data"
                n390 = xnode "FPGA I/O Node"("Connector1/DIO15"=TRUE) -> ()  [unwired: 1 in, 1 out]
              }
            }
          }
        }
      }
    }
  }
  n391 = while "Control APD data integration - stream to host" {
    shift-right: [w2111] -> _
    shift-left: w1 -> [w2116]
    stop <- FALSE stop-if-true
    n392 = flat-sequence {
      tunnel: w2116 -> [w2118]
      tunnel: [w2119] -> w2114
      tunnel: [w2118] -> w2112
      tunnel: [w2127] -> w2115
      tunnel: w2114 -> [w2127]
      tunnel: [w2126] -> w2113
      tunnel: w2112 -> [w2126]
      tunnel: [w2125] -> w2110
      tunnel: [w2124] -> w2109
      tunnel: [w2151] -> w2111
      tunnel: w2115 -> [w2176]
      tunnel: w2113 -> [w2173]
      tunnel: w2110 -> [w2144]
      tunnel: w2109 -> [w2143]
      frame #0 {
        n393 = call "Loop Timer6"("Count(Ticks)"=w2118) -> ("Tick Count(Ticks)"=w2119:u32)
      }
      frame #1 {
        n394 = flat-sequence {
          tunnel: [w2128] -> w2123
          tunnel: w2123 -> [w2131]
          tunnel: [w2133] -> w2122
          tunnel: [w2132] -> w2121
          tunnel: [w2131] -> w2120
          tunnel: [w2139] -> w2124
          tunnel: [w2140] -> w2125
          tunnel: w2122 -> [w2140]
          tunnel: w2121 -> [w2139]
          tunnel: w2120 -> [w2138]
          frame #0 {
            n395 = feedback #32(FALSE) -> (w2129:bool)
            "APD out state" <- w2129
            n396 = Not(x=w2129) -> (.not. x?=w2128:bool)
          }
          frame #1 {
            n397 = local read "APD 1 Counts 1"() -> (w2137:u32)
            n398 = local read "APD 1 Counts 0"() -> (w2136:u32)
            n399 = local read "APD 2 Counts 1"() -> (w2135:u32)
            n400 = local read "APD 2 Counts 0"() -> (w2134:u32)
            n401 = Select(t=w2137, s=w2131, f=w2136) -> (s? t:f=w2133:u32)
            n402 = Select(t=w2135, s=w2131, f=w2134) -> (s? t:f=w2132:u32)
          }
          frame #2 {
            n403 = case shown="False" w2138 {
              frame #0 {
                w2141 = u32 0 ("APD 1 Counts 0")
                n404 = local write "APD 1 Counts 0"(w2141) -> ()
                n405 = local write "APD 2 Counts 0"(w2141) -> ()
              }
              frame #1 {
                w2142 = u32 0 ("APD 1 Counts 1")
                n406 = local write "APD 1 Counts 1"(w2142) -> ()
                n407 = local write "APD 2 Counts 1"(w2142) -> ()
              }
            }
          }
        }
      }
      frame #2 {
        n408 = feedback #33(w2176) -> (w2175:u32)
        n409 = Subtract(x=w2176, y=w2175) -> (x-y=w2174:u32)
        n410 = Subtract(x=w2174, y=w2173) -> (x-y=w2167:u32)
        n411 = case shown="True" "APD to FIFO" {
          tunnel: w2144 -> [_ w2203]
          tunnel: w2143 -> [_ w2201]
          frame #0 {
          }
          frame #1 {
            n412 = flat-sequence {
              tunnel: 0 ("Timeout") -> [w2205]
              tunnel: w2203 -> [w2206]
              tunnel: [w2205] -> w2202
              tunnel: w2202 -> [w2233]
              tunnel: w2201 -> [w2232]
              frame #0 {
                n413 = xnode ("FIFO Write")("Element"=w2206, "Timeout"=w2205) -> ()  [unwired: 1 in, 2 out]
              }
              frame #1 {
                n414 = xnode ("FIFO Write")("Element"=w2232, "Timeout"=w2233) -> ()  [unwired: 1 in, 2 out]
              }
            }
          }
        }
        n415 = Subtract(x="APD Acq Rate Count", y=w2167) -> (x-y=w2152:u32)
        n416 = Greater?(x=w2167, y=u32 0) -> (0:w2169:bool)
        "APD Acq Late?" <- w2169
        n417 = feedback #34(u32 0) -> (w2171:u32)
        n418 = Increment(x=w2171) -> (x+1=w2170:u32)
        n419 = Select(t=w2170, s=w2169, f=w2171) -> (s? t:f=w2168:u32)
        "APD Acq Late Counter" <- w2168
        n420 = Boolean To (0,1)(Boolean="+ phase (APD Acq)") -> (0, 1=w2148:i16)
        n421 = Multiply(x=w2148, y="Phase Count Adjustment (APD Acq)") -> (x*y=w2145:i16)
        n422 = Add(x=w2152, y=w2145) -> (x+y=w2151:u32)
        n423 = feedback #35(i16 0) -> (w2150:i16)
        n424 = Subtract(x=w2150, y=w2145) -> (x-y=w2147:i16)
        "APD Acq Relative Phase" <- w2147
        n425 = To Word Integer(number=w2144) -> (16bit integer=w2160:i16)
        n426 = To Word Integer(number=w2143) -> (16bit integer=w2161:i16)
        n427 = Multiply(x="APD 1 AO scale factor", y=w2160) -> (x*y=w2159:i16)
        n428 = Multiply(x="APD 2 AO scale factor", y=w2161) -> (x*y=w2158:i16)
        n429 = Add(x="APD 1 AO offset", y=w2159) -> (x+y=w2157:i16)
        n430 = Add(x=w2158, y="APD 2 AO offset") -> (x+y=w2155:i16)
        n431 = xnode "FPGA I/O Node"("Connector0/AO6"=w2157, "Connector0/AO7"=w2155) -> ()  [unwired: 2 in, 2 out]
      }
    }
  }
  n432 = timed-loop "RF box board DIO control: control bits" {
    timing: w4 -> [_]
    timing-out: [_] -> w3
    tunnel: [w2259] -> _
    tunnel: w1 -> [w2259]
    stop <- FALSE stop-if-true
    n433 = xnode "FPGA I/O Node"("Connector1/DIO16"="RD", "Connector1/DIO17"="PMODE", "Connector1/DIO18"="OSK Bd 1", "Connector1/DIO19"="Reset Bd 1", "Connector1/DIO28"="OSK Bd 2", "Connector1/DIO29"="Reset Bd 2") -> ()  [unwired: 6 in, 6 out]
  }
  n434 = while "Green fluorescent laser interlacing (DO to IA 532 nm AOM ME amp)." {
    shift-right: [w2350] -> _
    shift-left: w1 -> [w2355]
    shift-right: [w2349] -> _
    shift-left: FALSE -> [w2347]
    stop <- FALSE stop-if-true
    n435 = flat-sequence {
      tunnel: w2355 -> [w2358]
      tunnel: [w2359] -> w2353
      tunnel: [w2358] -> w2351
      tunnel: [w2357] -> w2348
      tunnel: w2347 -> [w2357]
      tunnel: [w2362] -> w2354
      tunnel: w2353 -> [w2362]
      tunnel: [w2361] -> w2352
      tunnel: w2351 -> [w2361]
      tunnel: w2348 -> [w2360]
      tunnel: [w2402] -> w2350
      tunnel: w2354 -> [w2429]
      tunnel: w2352 -> [w2426]
      tunnel: [w2412] -> w2349
      frame #0 {
        n436 = call "Loop Timer4"("Count(Ticks)"=w2358) -> ("Tick Count(Ticks)"=w2359:u32)
      }
      frame #1 {
        n437 = xnode "FPGA I/O Node"("Connector1/DIO37"=w2360, "Connector1/DIO38"=w2360, "Connector1/DIO39"=w2360) -> ()  [unwired: 3 in, 3 out]
      }
      frame #2 {
        n438 = feedback #36(w2429) -> (w2428:u32)
        n439 = Subtract(x=w2429, y=w2428) -> (x-y=w2427:u32)
        n440 = Subtract(x=w2427, y=w2426) -> (x-y=w2418:u32)
        n441 = Greater?(x=w2418, y=u32 0) -> (0:w2422:bool)
        "GI Late?" <- w2422
        n442 = Boolean To (0,1)(Boolean="+ phase (GI)") -> (0, 1=w2407:i16)
        n443 = Multiply(x=w2407, y="Phase count adjustment (GI)") -> (x*y=w2404:i16)
        n444 = feedback #37(u32 0) -> (w2424:u32)
        n445 = Increment(x=w2424) -> (x+1=w2423:u32)
        n446 = Select(t=w2423, s=w2422, f=w2424) -> (s? t:f=w2421:u32)
        "GI Late Counter" <- w2421
        n447 = feedback #38(i16 0) -> (w2405:i16)
        n448 = Subtract(x=w2405, y=w2404) -> (x-y=w2403:i16)
        "GI Relative phase" <- w2403
        n449 = feedback #39(TRUE) -> (w2415:bool)
        n450 = case shown="2" "Operating Mode" {
          tunnel: [TRUE FALSE w2435] -> w2412
          tunnel: w2415 -> [_ _ w2432]
          frame #0 {
          }
          frame #1 {
          }
          frame #2 {
            n451 = Not(x=w2432) -> (.not. x?=w2434:bool)
            n452 = Select(t=w2434, s="Invert GI", f=w2432) -> (s? t:f=w2435:bool)
          }
        }
        n453 = Not(x=w2415) -> (.not. x?=w2411:bool)
        n454 = Select(t="Green interlace ON count", s=w2411, f="Green interlace OFF count") -> (s? t:f=w2417:u32)
        n455 = Subtract(x=w2417, y=w2418) -> (x-y=w2408:u32)
        n456 = Add(x=w2408, y=w2404) -> (x+y=w2402:u32)
      }
    }
  }
  n457 = while "Green fluorescent laser interlacing (Current to IA 532 nm AOM ME amp)." {
    shift-right: [w2441] -> _
    shift-left: w1 -> [w2444]
    shift-right: [w2438] -> _
    shift-left: w1 -> [w2436]
    stop <- FALSE stop-if-true
    n458 = flat-sequence {
      tunnel: w2444 -> [w2447]
      tunnel: [w2448] -> w2443
      tunnel: [w2447] -> w2442
      tunnel: [w2446] -> w2437
      tunnel: w2436 -> [w2446]
      tunnel: [w2451] -> w2440
      tunnel: w2443 -> [w2451]
      tunnel: [w2450] -> w2439
      tunnel: w2442 -> [w2450]
      tunnel: w2437 -> [w2449]
      tunnel: [w2464] -> w2441
      tunnel: [w2482] -> w2438
      tunnel: w2440 -> [w2501]
      tunnel: w2439 -> [w2498]
      frame #0 {
        n459 = call "Loop Timer10"("Count(Ticks)"=w2447) -> ("Tick Count(Ticks)"=w2448:u32)
      }
      frame #1 {
        n460 = xnode "FPGA I/O Node"("Chassis2/Mod4/AO0"=w2449) -> ()  [unwired: 1 in, 1 out]
      }
      frame #2 {
        n461 = Subtract(x="Green interlace OFF count 2", y="Green int current ON count adj") -> (x-y=w2474:u32)
        n462 = feedback #40(w2501) -> (w2500:u32)
        n463 = Add(x="Green int current ON count adj", y="Green interlace ON count 2") -> (x+y=w2475:u32)
        n464 = Subtract(x=w2501, y=w2500) -> (x-y=w2499:u32)
        n465 = Subtract(x=w2499, y=w2498) -> (x-y=w2490:u32)
        n466 = Greater?(x=w2490, y=u32 0) -> (0:w2494:bool)
        "GI Late? 2" <- w2494
        n467 = Boolean To (0,1)(Boolean="+ phase (GI) 2") -> (0, 1=w2470:i16)
        n468 = Multiply(x=w2470, y="Phase count adjustment (GI) 2") -> (x*y=w2466:i16)
        n469 = feedback #41(u32 0) -> (w2496:u32)
        n470 = Increment(x=w2496) -> (x+1=w2495:u32)
        n471 = Select(t=w2495, s=w2494, f=w2496) -> (s? t:f=w2493:u32)
        "GI Late Counter 2" <- w2493
        n472 = feedback #42(i16 0) -> (w2467:i16)
        n473 = Subtract(x=w2467, y=w2466) -> (x-y=w2465:i16)
        "GI Relative phase 2" <- w2465
        n474 = feedback #43(TRUE) -> (w2487:bool)
        n475 = case shown="2" "Operating Mode 2" {
          tunnel: [TRUE FALSE w2518] -> w2476
          tunnel: w2487 -> [_ _ w2515]
          frame #0 {
          }
          frame #1 {
          }
          frame #2 {
            n476 = Not(x=w2515) -> (.not. x?=w2517:bool)
            n477 = Select(t=w2517, s="Invert GI 2", f=w2515) -> (s? t:f=w2518:bool)
          }
        }
        n478 = And(x=w2476, y="Green FB On/Off") -> (x .and. y?=w2477:bool)
        n479 = case shown="True" w2477 {
          tunnel: "Current Out" -> [w2502 _]
          tunnel: [w2502 w2507] -> w2481
          frame #0 {
          }
          frame #1 {
            n480 = local read "Green FB Sum"() -> (w2503:i16)
            n481 = call "Slower PID.vi"("process variable"=w2503, "reset?"="Green FB Reset", "setpoint"="Green FB Setpoint", "PID gains (x 2^8)"="Green FB Gains", "output range"=cluster{"output high":i16, "output low":i16} {"output high"=32767, "output low"=-32768} ("Green FB output range")) -> ("output"=w2511:i16)  [unwired: 10 out]
            n482 = To Long Integer(number=w2511) -> (32bit integer=w2504:i32)
            n483 = Add(x=w2504, y=32768) -> (x+y=w2506:i32)
            n484 = To Unsigned Word Integer(number=w2506) -> (unsigned 16bit integer=w2507:u16)
          }
        }
        n485 = Not(x=w2487) -> (.not. x?=w2484:bool)
        n486 = Select(t=w2475, s=w2484, f=w2474) -> (s? t:f=w2489:u32)
        n487 = Subtract(x=w2489, y=w2490) -> (x-y=w2468:u32)
        n488 = Add(x=w2468, y=w2466) -> (x+y=w2464:u32)
        n489 = Boolean To (0,1)(Boolean=w2476) -> (0, 1=w2483:i16)
        n490 = To Unsigned Word Integer(number=w2483) -> (unsigned 16bit integer=w2480:u16)
        n491 = Multiply(x=w2480, y=w2481) -> (x*y=w2482:u16)
      }
    }
  }
  n492 = while "Green excitation laser feedback measurement" {
    shift-right: [w2519] -> _
    shift-left: w1 -> [w2524]
    stop <- FALSE stop-if-true
    n493 = flat-sequence {
      tunnel: w2524 -> [w2526]
      tunnel: [w2527] -> w2522
      tunnel: [w2526] -> w2520
      tunnel: [w2534] -> w2523
      tunnel: w2522 -> [w2534]
      tunnel: [w2533] -> w2521
      tunnel: w2520 -> [w2533]
      tunnel: [w2610] -> w2519
      tunnel: w2523 -> [w2628]
      tunnel: w2521 -> [w2625]
      frame #0 {
        n494 = call "Loop Timer9"("Count(Ticks)"=w2526) -> ("Tick Count(Ticks)"=w2527:u32)
      }
      frame #1 {
        n495 = xnode "FPGA I/O Node"("Connector1/DIO35"=TRUE) -> ("Chassis2/Mod1/AI0"=w2532:i16, "Chassis2/Mod1/AI1"=w2531:i16, "Chassis2/Mod1/AI2"=w2528:i16)  [unwired: 4 in, 4 out]
        "Green FB Sum" <- w2528
        n496 = Bundle("Chassis2/Mod1/AI0"=w2532, "Chassis2/Mod1/AI1"=w2531, "Chassis2/Mod1/AI2"=w2528) -> (→"Green FB Signals":T14)  [unwired: 1 out]
      }
      frame #2 {
        n497 = feedback #44(w2628) -> (w2627:u32)
        n498 = Subtract(x=w2628, y=w2627) -> (x-y=w2626:u32)
        n499 = xnode "FPGA I/O Node"("Connector1/DIO35"=FALSE) -> ()  [unwired: 1 in, 1 out]
        n500 = Subtract(x=w2626, y=w2625) -> (x-y=w2619:u32)
        n501 = Subtract(x="Green FB Count", y=w2619) -> (x-y=w2614:u32)
        n502 = Greater?(x=w2619, y=u32 0) -> (0:w2621:bool)
        "Green FB Late?" <- w2621
        n503 = Boolean To (0,1)(Boolean="+ phase (Green FB)") -> (0, 1=w2612:i16)
        n504 = Multiply(x=w2612, y="Phase count adjustment (Green FB)") -> (x*y=w2607:i16)
        n505 = feedback #45(u32 0) -> (w2623:u32)
        n506 = Increment(x=w2623) -> (x+1=w2622:u32)
        n507 = Select(t=w2622, s=w2621, f=w2623) -> (s? t:f=w2620:u32)
        "Green Late Counter" <- w2620
        n508 = Add(x=w2614, y=w2607) -> (x+y=w2610:u32)
        n509 = feedback #46(i16 0) -> (w2609:i16)
        n510 = Subtract(x=w2609, y=w2607) -> (x-y=w2608:i16)
        "Green FB Relative Phase" <- w2608
      }
    }
  }
  n511 = while "Control Additional IO (Green laser flip mount)" {
    stop <- FALSE stop-if-true
    n512 = xnode "FPGA I/O Node"("Connector0/DIO3"="Green Filter Flipper", "Connector0/DIO2"="Connector0/DIO9", "Connector1/DIO32"="Connector1/DIO32", "Connector1/DIO33"="Connector1/DIO33", "Connector1/DIO34"="Connector1/DIO34", "Chassis2/Mod4/AO1"="Chassis2/Mod4/AO1") -> ()  [unwired: 6 in, 6 out]
    n513 = call "Loop Timer2"("Count(Ticks)"="Extra DO Counts") -> ()  [unwired: 1 out]
  }
  n514 = node-c288(w3) -> ()
